vi "NI VeriStand - Remove Multiple Custom Device Items.vi"(7 "Skip action VI on delete (F)":bool, 8 "error in (no error)":errorcluster, 10 "Force Delete (F)":bool, 11 "Item Refs in":T1[](array[typedef]) format="%.0x") -> (0 "error out":errorcluster, 3 "Deleted?":bool)   [LabVIEW 2026, in "Custom Devices Storage.lvlib"]
uses:
  Custom Devices Storage.lvlib
  <vilib>/NI VeriStand/Custom Device API/Custom Device Item Ref.ctl
  <vilib>/NI VeriStand/Custom Device API/Custom Device API.lvlib
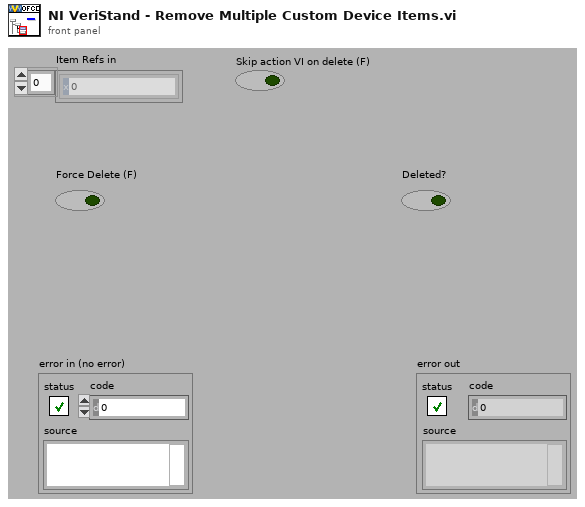
[diagram p1: front panel]
types:
  T1 = typedef "Custom Device API.lvlib/Custom Device Item Ref.ctl" = u64
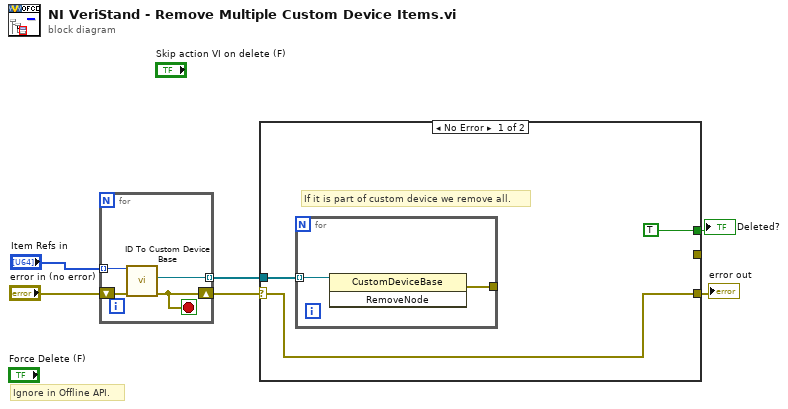
[diagram p0: block diagram]
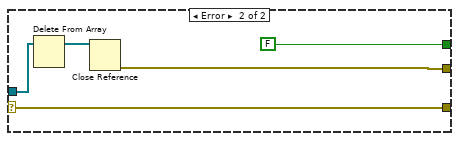
[diagram p2: hidden frame]
diagram:
  # "Ignore in Offline API."
  n1 = for {
    tunnel: "Item Refs in" -> [w10] mode=indexing
    shift-right: [w8] -> w4
    shift-left: "error in (no error)" -> [w9]
    tunnel: [w7] -> w1 mode=indexing
    stop <- w8 stop-if-true
    n2 = call "ID To Custom Device Base.vi"("error in (no error)"=w9, "ID in"=w10) -> ("error out"=w8:errorcluster, "BaseNode"=w7:refnum<k39>)  [unwired: 7 in, 1 out]
  }
  n3 = case shown="No Error" w4 {
    selector: w4 -> [w11 w20]
    tunnel: [w11 w20] -> w3
    tunnel: [TRUE FALSE] -> w2
    tunnel: w1 -> [w13 w18]
    tunnel: [_ w16] -> _
    frame No Error {
      # "If it is part of custom device we remove all."
      n4 = for {
        tunnel: w13 -> [w15] mode=indexing
        tunnel: [w14] -> _
        n5 = invoke class="CustomDeviceBase" method="RemoveNode"(reference=w15) -> (error out=w14:errorcluster)  [unwired: 2 in, 2 out]
      }
    }
    frame Error {
      n6 = Delete From Array(array=w18) -> (array with subset deleted=w17:refnum<k39>[])  [unwired: 2 in, 1 out]
      n7 = Close Reference(reference=w17) -> (error out=w16:errorcluster)  [unwired: 1 in]
    }
  }
  "error out" <- w3
  "Deleted?" <- w2
